vi "Destroy.vi"(8 "error in (no error)":errorcluster, 11 "ClientPool in":refnum<class "gRPC Client Pool.lvclass">) -> (0 "error out":errorcluster, 3 "ClientPool out":refnum<class "gRPC Client Pool.lvclass">)   [LabVIEW 2020, in "MeasurementLink gRPC Utilities.lvlib" / "gRPC Client Pool.lvclass"]
uses:
  gRPC Client Pool.lvclass
  gRPC Client Pool.lvclass/gRPC Client Pool.ctl
  <vilib>/gRPC/LabVIEW gRPC Library/Shared/grpcId.ctl
  MeasurementLink Discovery Client/MeasurementLink Discovery Client.lvlib
  MeasurementLink Pin Map Client/MeasurementLink Pin Map Client.lvlib
  MeasurementLink Session Management Client/MeasurementLink Session Management Client.lvlib
  <vilib>/gRPC/LabVIEW gRPC Library/grpc-lvsupport-release.lvlib
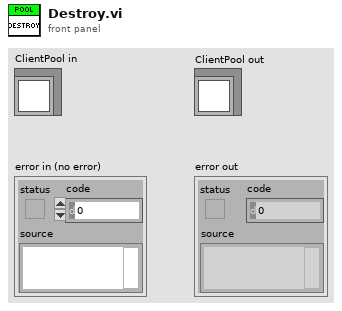
[diagram p1: front panel]
types:
  T1 = typedef "grpc-lvsupport-release.lvlib/grpcId.ctl" = u64
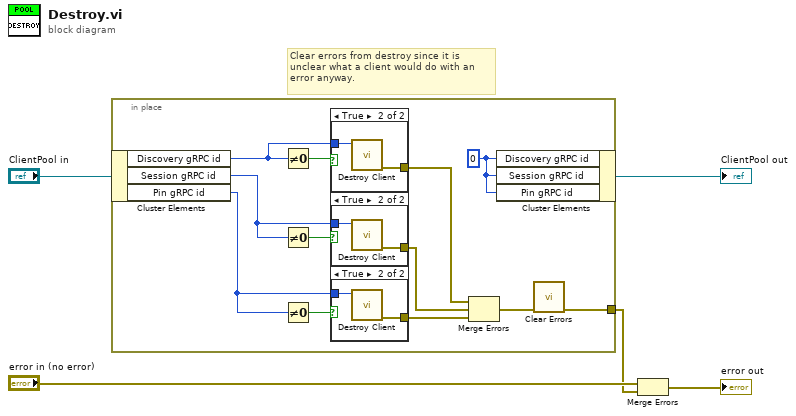
[diagram p0: block diagram]
diagram:
  # "Clear errors from destroy since it is \nunclear what a client would do with an\nerror anyway."
  n1 = in-place {
    in-place-border: [w6] -> w1
    w17 = T1 0 ("Discovery gRPC id")
    n2 = in-place-cluster #1("ClientPool in") -> ("Discovery gRPC id"=w13:T1, "Session gRPC id"=w12:T1, "Pin gRPC id"=w11:T1)
    n3 = Not Equal To 0?(x=w13) -> (x != 0?=w16:bool)
    n4 = Not Equal To 0?(x=w12) -> (x != 0?=w14:bool)
    n5 = Not Equal To 0?(x=w11) -> (x != 0?=w15:bool)
    n6 = case shown="True" w16 {
      tunnel: w13 -> [_ w23]
      tunnel: [_ w22] -> w10
      frame False {
      }
      frame True {
        n7 = call "Destroy Client.vi"("gRPC ID"=w23) -> ("error out"=w22:errorcluster)  [unwired: 10 in]
      }
    }
    n8 = case shown="True" w14 {
      tunnel: w12 -> [_ w21]
      tunnel: [_ w20] -> w9
      frame False {
      }
      frame True {
        n9 = call "Destroy Client.vi"("gRPC ID"=w21) -> ("error out"=w20:errorcluster)  [unwired: 10 in]
      }
    }
    n10 = case shown="True" w15 {
      tunnel: w11 -> [_ w19]
      tunnel: [_ w18] -> w8
      frame False {
      }
      frame True {
        n11 = call "Destroy Client.vi"("gRPC ID"=w19) -> ("error out"=w18:errorcluster)  [unwired: 10 in]
      }
    }
    n12 = Merge Errors(w10, w9, w8) -> (w7:errorcluster)
    n13 = in-place-cluster #1("Discovery gRPC id"=w17, "Session gRPC id"=w17, "Pin gRPC id"=w17) -> (→"ClientPool out":refnum<class "gRPC Client Pool.lvclass">)
    n14 = call <vilib>:"Clear Errors.vi"("error in (no error)"=w7) -> ("error out"=w6:errorcluster)  [unwired: 5 in, 1 out]
  }
  n15 = Merge Errors("error in (no error)", w1) -> (→"error out":errorcluster)
